vi "Send Update UE.vi"(8 "error in (no error)":errorcluster, 9 "Payload":variant, 10 "Update Message":string, 11 "Process in":refnum<class "Process.lvclass">) -> (0 "error out":errorcluster, 3 "Process out":refnum<class "Process.lvclass">)   [LabVIEW 2019, in "TimingDRV Engine.lvlib" / "Process.lvclass"]
uses:
  Process.lvclass
  TypeDefs/Update.ctl
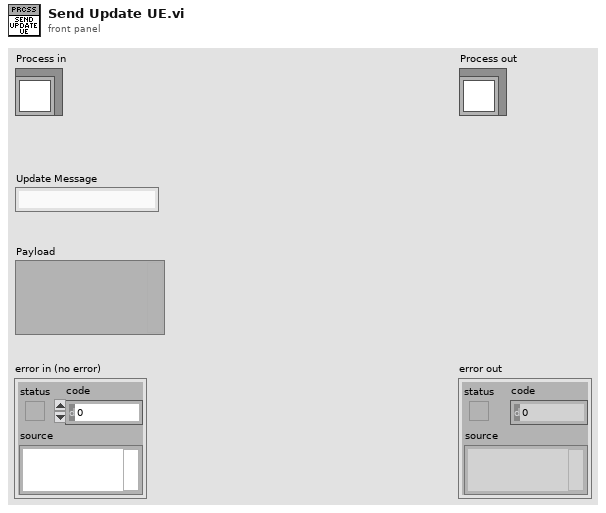
[diagram p1: front panel]
types:
  T1 = typedef "TimingDRV Engine.lvlib/Process.lvclass/Update.ctl" = cluster{"Update Message":string, "Payload":variant}
  T2 = typedef "TimingDRV Engine.lvlib/Process.lvclass/Process Lookup.ctl" = cluster{"Process ID":string, "MessageQ":refnum<queue>, "Update UE":refnum<user-event>}
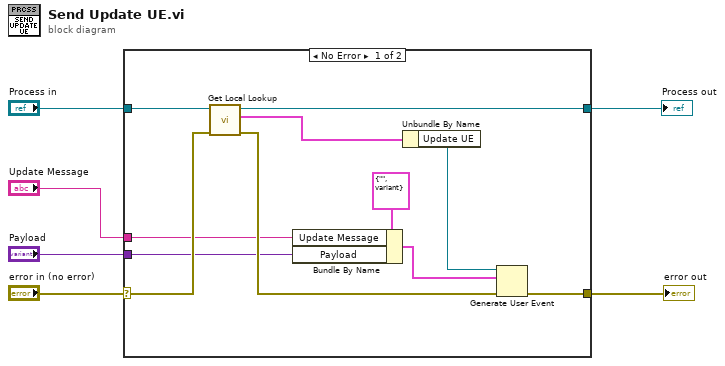
[diagram p0: block diagram]
diagram:
  n1 = case shown="No Error" "error in (no error)" {
    selector: "error in (no error)" -> [w12 w19]
    tunnel: [w9 w19] -> w5
    tunnel: [w13 w18] -> w3
    tunnel: "Process in" -> [w14 w18]
    tunnel: "Update Message" -> [w8 _]
    tunnel: "Payload" -> [w7 _]
    frame No Error {
      n2 = call-dynamic "Get Local Lookup.vi"("error in (no error)"=w12, "Process in"=w14) -> ("error out"=w15:errorcluster, "Process Lookup"=w17:T2, "Process out"=w13:refnum<class "Process.lvclass">)  [unwired: 7 in]
      n3 = Bundle By Name(cluster=T1 {"Update Message"="", "Payload"=variant} ("event data"), "Update Message"=w8, "Payload"=w7) -> (w10:T1)
      n4 = Unbundle By Name(w17) -> ("Update UE"=w16:refnum<user-event>)
      n5 = Generate User Event(user event=w16, event data cluster=w10, error in=w15) -> (error out=w9:errorcluster)  [unwired: 1 in, 1 out]
    }
    frame Error {
    }
  }
  "error out" <- w5
  "Process out" <- w3
